vi "5.tuning-pid-controller.vi"() -> ()   [LabVIEW 2011]
panel:
  in  "kd":dbl
  in  "ki":dbl min=0.0 max=100.0 step=0.01
  in  "kp":dbl min=0.0 max=1000.0 step=0.1
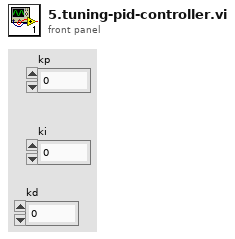
[diagram p1: front panel]
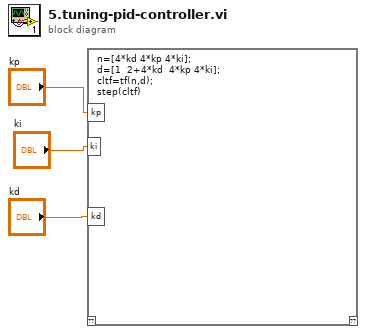
[diagram p0: block diagram]
diagram:
  n1 = script code="n=[4*kd 4*kp 4*ki];\nd=[1  2+4*kd  4*kp 4*ki];\ncltf=tf(n,d);\nstep(cltf)"("kp"="kp", "ki"="ki", "kd"="kd") -> ()  [unwired: 1 in, 1 out]
